vi "Clone.vi"(8 "error in (no error)":errorcluster, 11 "Config Manager in":refnum<class "Config Manager.lvclass">) -> (0 "error out":errorcluster, 2 "Cloned Manager":refnum<class "Config Manager.lvclass">, 3 "Config Manager out":refnum<class "Config Manager.lvclass">)   [LabVIEW 2020, in "CDM-Config.lvlib" / "Config Manager.lvclass"]
uses:
  Config Manager.lvclass
  Config Manager.lvclass/Config Manager.ctl
  Config Element/Config Element.lvclass
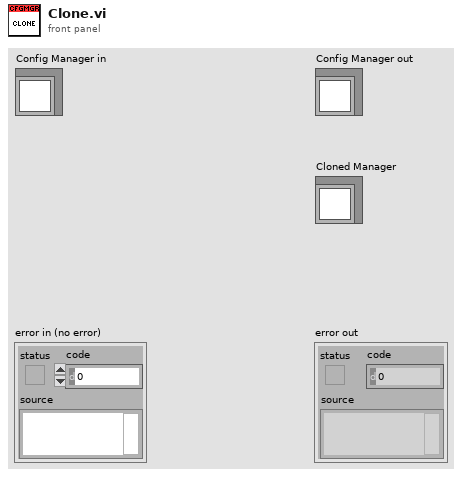
[diagram p1: front panel]
types:
  T1 = typedef "CDM-Config.lvlib/Config Manager.lvclass/Ref Data.ctl" = cluster{"Elements":refnum<class "Config Element.lvclass">[], "Hierarchy Map":map{string[], i32}, "Element Map":map{refnum<class "Config Element.lvclass">, i32}}
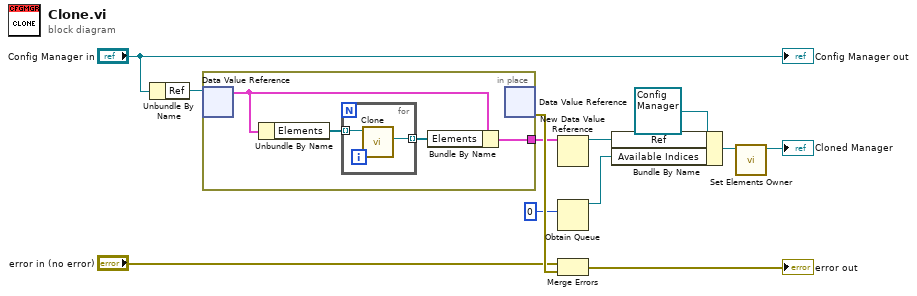
[diagram p0: block diagram]
diagram:
  n1 = Unbundle By Name("Config Manager in") -> ("Ref"=w9:refnum<data-value>)
  n2 = in-place {
    in-place-border: [w13] -> w8
    n3 = in-place-dvr #1(w9) -> (w15:T1)  [unwired: 1 out]
    n4 = Unbundle By Name(w15) -> ("Elements"=w16:refnum<class "Config Element.lvclass">[])
    n5 = for {
      tunnel: [w18] -> w14 mode=indexing
      tunnel: w16 -> [w17] mode=indexing
      n6 = call "Clone.vi"("Config Element in"=w17) -> ("Cloned Element"=w18:refnum<class "Config Element.lvclass">)  [unwired: 8 in, 2 out]
    }
    n7 = Bundle By Name(cluster=w15, "Elements"=w14) -> (w13:T1)
    n8 = in-place-dvr #1() -> (w12:errorcluster)  [unwired: 1 in, 1 out]
  }
  n9 = New Data Value Reference(data value=w8) -> (data value reference=w5:refnum<data-value>)  [unwired: 1 in, 1 out]
  n10 = Obtain Queue(element data type=0) -> (queue out=w4:refnum<queue>)  [unwired: 4 in, 2 out]
  n11 = Merge Errors("error in (no error)", w12) -> (→"error out":errorcluster)
  n12 = Bundle By Name(cluster=refnum<class "Config Manager.lvclass"> refnum ("Cloned Manager"), "Ref"=w5, "Available Indices"=w4) -> (w3:refnum<class "Config Manager.lvclass">)
  n13 = call "Set Elements Owner.vi"("Config Manager in"=w3) -> ("Config Manager out"=→"Cloned Manager":refnum<class "Config Manager.lvclass">)  [unwired: 9 in, 1 out]
  "Config Manager out" <- "Config Manager in"
